vi "rad_Check Image RT-INI For AutoRun.vi"(8 "error in (no error)":errorcluster, 9 "target settings":T1={"Hostname"="", "Serial number"="", "Product name"="", "Product code"=0, "System status"="", "Credential type"=enum."None/Unlocked", "User added?"=FALSE, "Primary NIC"={"MAC address"="", "IP Address Request Mode"=2, "IP address"="", "Subnet mask"="", "Gateway"="", "DNS server"=""}} {"Primary NIC"."IP Address Request Mode" items=["Static"=1, "DHCP/Link-Local"=2, "Link-Local Only"=4, "DHCP Only"=8]}, 11 "temp folder":path) -> (0 "error out":errorcluster, 2 "Run at Startup?":bool, 3 "temp folder out":path)   [LabVIEW 2023]
uses:
  Targets/TypeDefs/rad_Target Information.ctl
  Targets/TypeDefs/rad_Target Network Settings.ctl
  <vilib>/Utility/config.llb/Read Key (Boolean).vi
  <vilib>/nisyscfg/Close (Hardware).vi
  <vilib>/nisyscfg/Close (System).vi
  <vilib>/Utility/config.llb/NI_LVConfig.lvlib
  <resource>/objmgr/nisysapi.rc
  <resource>/objmgr/nicriosae.rc
  <vilib>/nisyscfg/nisyscfg.lvlib
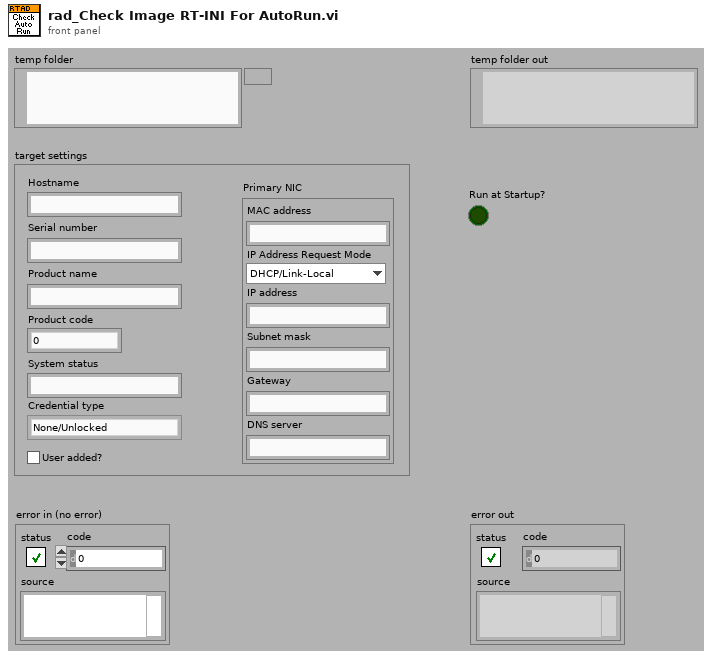
[diagram p1: front panel]
types:
  T1 = typedef "rad_Target Information.ctl" = cluster{"Hostname":string, "Serial number":string, "Product name":string, "Product code":i32, "System status":string, "Credential type":enum16{"None/Unlocked", "FTP Password", "NIAuth Credentials"}, "User added?":bool, "Primary NIC":T2}
  T2 = typedef "rad_Target Network Settings.ctl" = cluster{"MAC address":string, "IP Address Request Mode":i32, "IP address":string, "Subnet mask":string, "Gateway":string, "DNS server":string}
  T3 = enum16{"None/Unlocked", "FTP Password", "NIAuth Credentials"}
  T4 = typedef "NI_LVConfig.lvlib/Config Data RefNum.ctl" = refnum<k1>
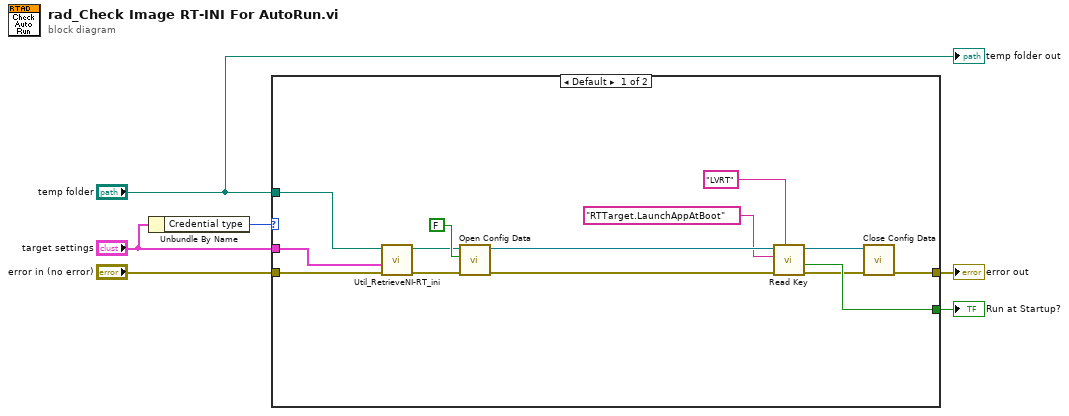
[diagram p0: block diagram]
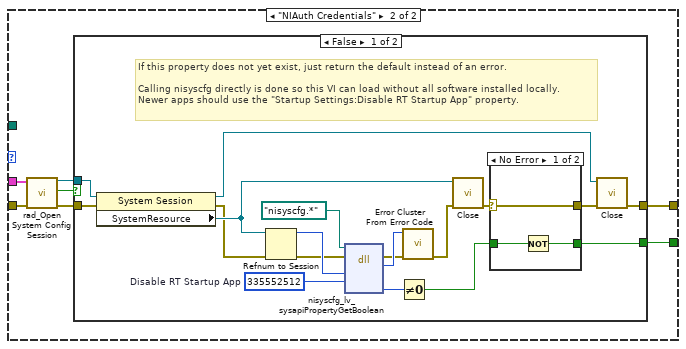
[diagram p2: hidden frame]
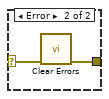
[diagram p3: hidden frame]
diagram:
  n1 = Unbundle By Name("target settings") -> ("Credential type"=w3:T3)
  n2 = case shown="Default" w3 {
    tunnel: [w17 w22] -> w6
    tunnel: [w14 w21] -> w5
    tunnel: "temp folder" -> [w11 _]
    tunnel: "target settings" -> [w7 w27]
    tunnel: "error in (no error)" -> [w9 w26]
    frame Default {
      n3 = call "Util_RetrieveNI-RT_ini.vi"("error in"=w9, "Target settings"=w7, "temp folder"=w11) -> ("error out"=w8:errorcluster, "Ini File Path"=w10:path)  [unwired: 7 in]
      n4 = call <vilib>:"Open Config Data.vi"("error in (no error)"=w8, "create file if necessary (T)"=FALSE, "configuration file path"=w10) -> ("error out"=w18:errorcluster, "refnum"=w19:T4)  [unwired: 6 in, 1 out]
      n5 = call-poly <vilib>:"Read Key.vi"("section"="LVRT", "error in (no error)"=w18, "key"="RTTarget.LaunchAppAtBoot", "refnum"=w19) -> ("error out"=w13:errorcluster, "value"=w17:bool, "refnum out"=w12:T4)  [unwired: 4 in, 1 out]
      n6 = call <vilib>:"Close Config Data.vi"("error in (no error)"=w13, "refnum"=w12) -> ("error out"=w14:errorcluster)  [unwired: 8 in, 1 out]
    }
    frame "NIAuth Credentials" {
      n7 = call "rad_Open System Config Session.vi"("error in (no error)"=w26, "Target settings"=w27) -> ("error out"=w23:errorcluster, "Cancelled"=w24:bool, "Session out"=w25:refnum<k21>)  [unwired: 6 in, 1 out]
      n8 = case shown="False" w24 {
        tunnel: w25 -> [w45 _]
        tunnel: w23 -> [w44 w51]
        tunnel: [w42 w51] -> w21
        tunnel: [w39 _] -> w22
        frame False {
          w37 = u32 335552512  # Disable RT Startup App
          # "If this property does not yet exist, just return the default instead of an error.\n\nCalling nisyscfg directly is done so this VI can load without all software installed locally.\nNewer apps should use the \"Startup Settings:Disable RT Startup App\" property."
          n9 = property class="System Session"(reference=w45, error in=w44) -> (reference out=w43:refnum<k21>, error out=w31:errorcluster, "SystemResource"=w32:refnum<k20>)
          n10 = Refnum to Session(4:w31, 7:w32) -> (0:w33:errorcluster, 3:w38:u64)
          n11 = dll-call lib="nisyscfg.dll" fn="nisyscfg_lv_sysapiPropertyGetBoolean"(path in=path "nisyscfg.*", error in=w33, "resource"=w38, "attribute"=w37) -> (error out=w34:errorcluster, "status"=w36:i32, "value"=w29:u8)  [unwired: 4 in, 1 out]
          n12 = Not Equal To 0?(x=w29) -> (x != 0?=w28:bool)
          n13 = call <vilib>:"Error Cluster From Error Code.vi"("error in (no error)"=w34, "error code (0)"=w36) -> ("error out"=w30:errorcluster)  [unwired: 2 in, 5 out]
          n14 = call-poly <vilib>:"Close.vi"("error in (no error)"=w30, "Resource in"=w32) -> ("error out"=w41:errorcluster)  [unwired: 9 in]
          n15 = case shown="No Error" w41 {
            selector: w41 -> [w48 w50]
            tunnel: [w48 w49] -> w40
            tunnel: [w47 _] -> w39
            tunnel: w28 -> [w46 _]
            frame No Error {
              n16 = Not(x=w46) -> (.not. x?=w47:bool)
            }
            frame Error {
              n17 = call <vilib>:"Clear Errors.vi"("error in (no error)"=w50) -> ("error out"=w49:errorcluster)  [unwired: 5 in, 1 out]
            }
          }
          n18 = call-poly <vilib>:"Close.vi"("error in (no error)"=w40, "Session in"=w43) -> ("error out"=w42:errorcluster)  [unwired: 9 in]
        }
        frame True {
        }
      }
    }
  }
  "Run at Startup?" <- w6
  "error out" <- w5
  "temp folder out" <- "temp folder"
